vi "to_xml.vi"(8 "error in":errorcluster, 11 "Camera Setup":T1={"Analog Gain (0-5)"=4, "Exposure Time"=0.01, "EM Gain (0-255)"=0, "Trigger Polarity"="ATP P", "External Trigger Mode"="ATP P", "Scan Speed"="EMD E", "External Trigger Source"="SSP H", "Scan Mode"="ESC B", "Super Pixel Binning\n(if enabled in Scan Mode)"="SMD N", "Camera Sub-array acquisition region\n(if enabled in scan mode)"={"Left"=0, "Top"=0, "Width"=0, "Height"=0}, "Use camera?"=FALSE, "# image buffers"=100, "shots per measurement"=100, "Force images to U16"=FALSE, "Low Light Sensitivity"="LLS 0", "cooling"="LLS 0", "fan"="LLS 0", "Frame Grabber acquisition region"={"Left"=0, "Top"=0, "Right"=0, "Bottom"=0}} {"Frame Grabber acquisition region"."Bottom" max=512 step=1; "Frame Grabber acquisition region"."Right" max=512 step=1; "Frame Grabber acquisition region"."Top" max=512 step=1; "Frame Grabber acquisition region"."Left" max=512 step=1; "shots per measurement" min=0 step=1; "# image buffers" min=0 step=1; "Camera Sub-array acquisition region\n(if enabled in scan mode)"."Height" min=16 max=512 step=16; "Camera Sub-array acquisition region\n(if enabled in scan mode)"."Width" min=16 max=512 step=16; "Camera Sub-array acquisition region\n(if enabled in scan mode)"."Top" max=496 step=16; "Camera Sub-array acquisition region\n(if enabled in scan mode)"."Left" max=496 step=16; "Analog Gain (0-5)" max=5 step=1}) -> (0 "error out":errorcluster, 3 "Camera Setup string":string)   [LabVIEW 2013, in "Hamamatsu_C9100-13.lvclass"]
doc: "Converts Hamamatsu C9100-13 camera settings to xml in the format:\n\n<Enable>%b</Enable>\n<AnalogGain>%u</AnalogGain>\n<FrameGrabberAcquisitionRegion columns=\"left, top, right, bottom\">%u %u %u %u</FrameGrabberAcquisitionRegion>\n<ExposureTime>%f</ExposureTime>\n<EMGain>%u</EMGain>\n<TriggerPolarity>%s</TriggerPolarity>\n<ExternalTriggerMode>%s</ExternalTriggerMode>\n<ScanSpeed>%s</ScanSpeed>\n<ExternalTriggerSource>%s</ExternalTriggerSource>\n<ScanMode>%s</ScanMode>\n<SuperPixelBinning>%s</SuperPixelBinning>\n<CameraSubArrayAcquisitionRegion columns=\"left, top, width, height\">%u %u %u %u</CameraSubArrayAcquisitionRegion>\n<NumberOfImageBuffers>%u</NumberOfImageBuffers>\n<RegionsOfInterest columns=\"Left, Top, Right Bottom\">\n%s</RegionsOfInterest>\n<BackgroundRegions columns=\"Left, Top, Right Bottom\">\n%s</BackgroundRegions>\n<ShotsPerMeasurement>%u</ShotsPerMeasurement>\n<PhotoelectronScaling>%f</PhotoelectronScaling>\n\nMTL 2013 Jan 1"
uses:
  Hamamatsu_C9100-13.lvclass
  camera_setup.ctl
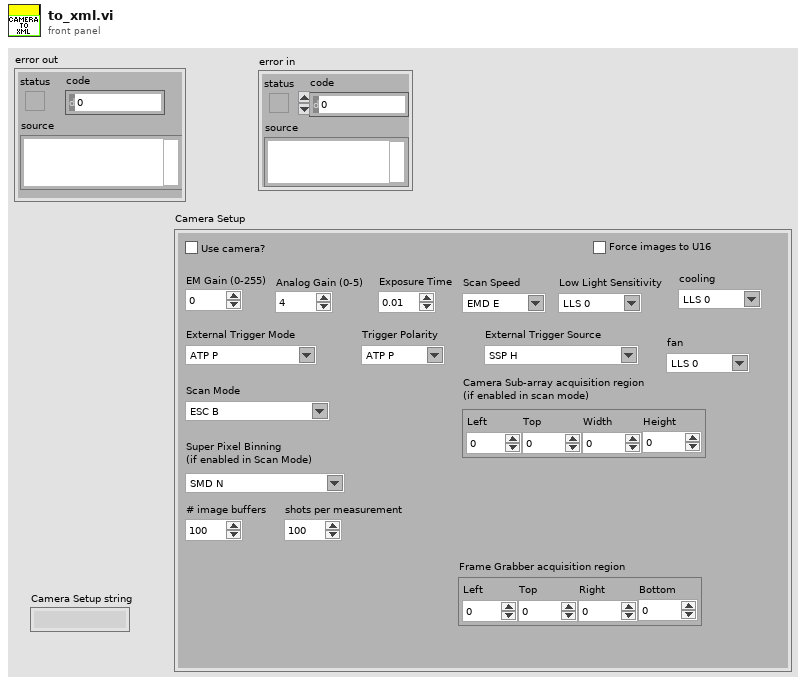
[diagram p1: front panel]
types:
  T1 = typedef "Hamamatsu_C9100-13.lvclass/camera_setup.ctl" = cluster{"Analog Gain (0-5)":u8, "Exposure Time":dbl, "EM Gain (0-255)":u8, "Trigger Polarity":string, "External Trigger Mode":string, "Scan Speed":string, "External Trigger Source":string, "Scan Mode":string, "Super Pixel Binning\n(if enabled in Scan Mode)":string, "Camera Sub-array acquisition region\n(if enabled in scan mode)":cluster{"Left":u16, "Top":u16, "Width":u16, "Height":u16}, "Use camera?":bool, "# image buffers":i32, "shots per measurement":i32, "Force images to U16":bool, "Low Light Sensitivity":string, "cooling":string, "fan":string, "Frame Grabber acquisition region":cluster{"Left":i32, "Top":i32, "Right":i32, "Bottom":i32}}
  T2 = cluster{"Left":u16, "Top":u16, "Width":u16, "Height":u16}
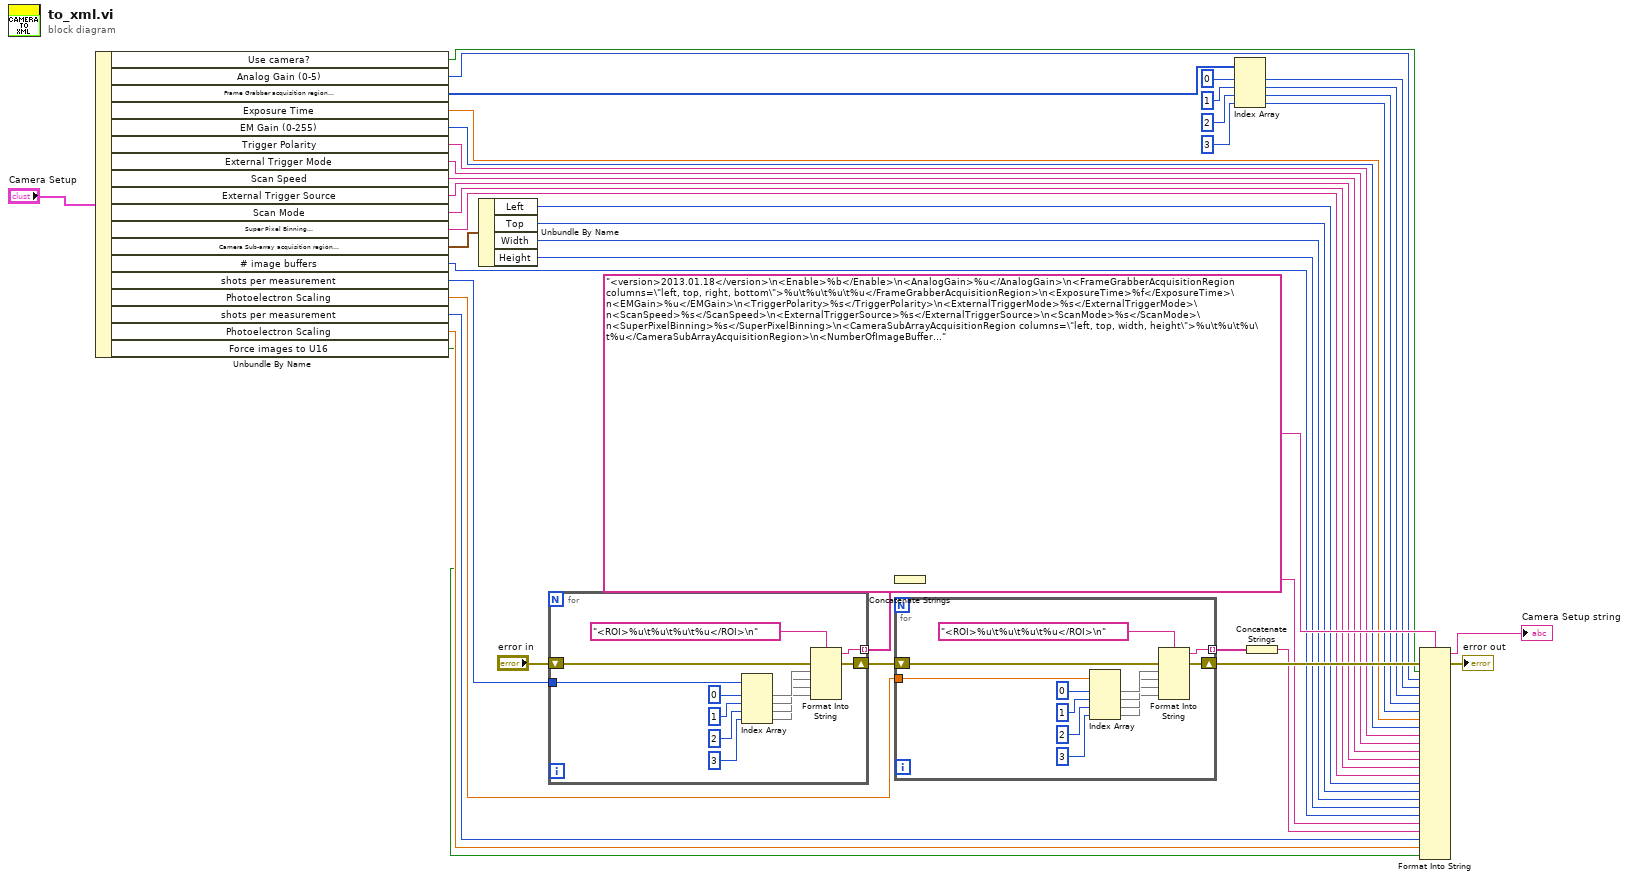
[diagram p0: block diagram]
diagram:
  n1 = Unbundle By Name("Camera Setup") -> ("Use camera?"=w7:bool, "Analog Gain (0-5)"=w8:u8, "Frame Grabber acquisition region\n(left, top, right, bottom)"=w6:i32[], "Exposure Time"=w27:dbl, "EM Gain (0-255)"=w26:u8, "Trigger Polarity"=w25:string, "External Trigger Mode"=w24:string, "Scan Speed"=w23:string, "External Trigger Source"=w22:string, "Scan Mode"=w21:string, "Super Pixel Binning\n(if enabled in Scan Mode)"=w20:string, "Camera Sub-array acquisition region\n(if enabled in scan mode)"=w37:T2, "# image buffers"=w15:i32, "shots per measurement"=w36:i32, "Photoelectron Scaling"=w35:dbl, "shots per measurement"=w14:i32, "Photoelectron Scaling"=w12:dbl, "Force images to U16"=w1:bool)
  n2 = Unbundle By Name(w37) -> ("Left"=w19:u16, "Top"=w18:u16, "Width"=w17:u16, "Height"=w16:u16)
  n3 = for {
    tunnel: w36 -> [w54]
    shift-right: [w43] -> w34
    shift-left: "error in" -> [w44]
    tunnel: [w42] -> w5 mode=indexing
    n4 = Index Array(array=w54, index #1=0 ("index"), index #2=1 ("index"), index #3=2 ("index"), index #4=3 ("index")) -> (element #1=w49, element #2=w48, element #3=w47, element #4=w46)
    n5 = Format Into String(format string="<ROI>%u\t%u\t%u\t%u</ROI>\n", error in=w44, w49, w48, w47, w46) -> (resulting string=w42:string, error out=w43:errorcluster)  [unwired: 1 in]
  }
  n6 = Concatenate Strings(w5) -> (w3:string)
  n7 = for {
    tunnel: w35 -> [w67]
    shift-right: [w55] -> w32
    shift-left: w34 -> [w56]
    tunnel: [w57] -> w4 mode=indexing
    n8 = Index Array(array=w67, index #1=0 ("index"), index #2=1 ("index"), index #3=2 ("index"), index #4=3 ("index")) -> (element #1=w62, element #2=w61, element #3=w60, element #4=w59)
    n9 = Format Into String(format string="<ROI>%u\t%u\t%u\t%u</ROI>\n", error in=w56, w62, w61, w60, w59) -> (resulting string=w57:string, error out=w55:errorcluster)  [unwired: 1 in]
  }
  n10 = Index Array(array=w6, index #1=0 ("index"), index #2=1 ("index"), index #3=2 ("index"), index #4=3 ("index")) -> (element #1=w31:i32, element #2=w30:i32, element #3=w29:i32, element #4=w28:i32)
  n11 = Concatenate Strings(w4) -> (w2:string)
  n12 = Format Into String(format string="<version>2013.01.18</version>\n<Enable>%b</Enable>\n<AnalogGain>%u</AnalogGain>\n<FrameGrabberAcquisitionRegion columns=\"left, top, right, bottom\">%u\t%u\t%u\t%u</FrameGrabberAcquisitionRegion>\n<ExposureTime>%f</ExposureTime>\n<EMGain>%u</EMGain>\n<TriggerPolarity>%s</TriggerPolarity>\n<ExternalTriggerMode>%s</ExternalTriggerMode>\n<ScanSpeed>%s</ScanSpeed>\n<ExternalTriggerSource>%s</ExternalTriggerSource>\n<ScanMode>%s</ScanMode>\n<SuperPixelBinning>%s</SuperPixelBinning>\n<CameraSubArrayAcquisitionRegion columns=\"left, top, width, height\">%u\t%u\t%u\t%u</CameraSubArrayAcquisitionRegion>\n<NumberOfImageBuffers>%u</NumberOfImageBuffers>\n<RegionsOfInterest columns=\"Left, Top, Right Bottom\">\n%s</RegionsOfInterest>\n<BackgroundRegions columns=\"Left, Top, Right Bottom\">\n%s</BackgroundRegions>\n<ShotsPerMeasurement>%u</ShotsPerMeasurement>\n<PhotoelectronScaling>%f</PhotoelectronScaling>\n<ForceImagesToU16>%b</ForceImagesToU16>", error in=w32, w7, w8, w31, w30, w29, w28, w27, w26, w25, w24, w23, w22, w21, w20, w19, w18, w17, w16, w15, w3, w2, w14, w12, w1) -> (resulting string=→"Camera Setup string":string, error out=→"error out":errorcluster)  [unwired: 1 in]
